vi "Error Converter (ErrCode or Status).vi"(7 "source":string, 10 "error code":i32, 11 "error in (no error)":errorcluster) -> (3 "error out":errorcluster)   [LabVIEW 2026, in "synnax_clib.lvlib"]
uses:
  synnax_clib.lvlib
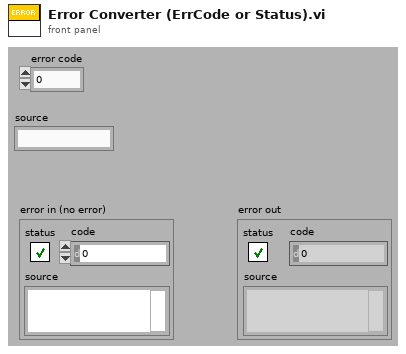
[diagram p1: front panel]
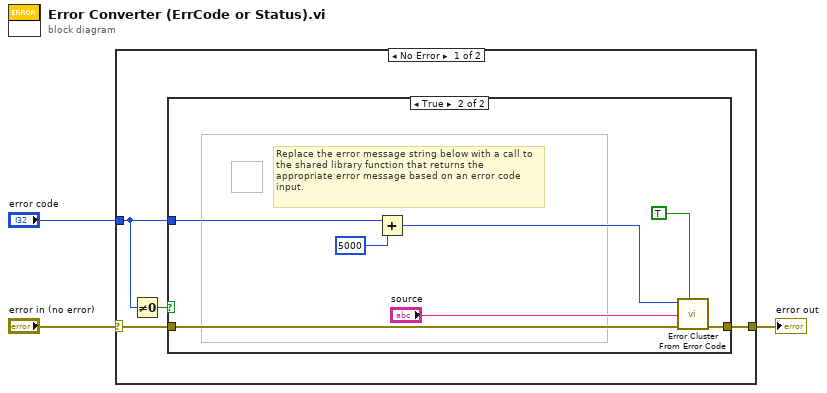
[diagram p0: block diagram]
diagram:
  n1 = case shown="No Error" "error in (no error)" {
    selector: "error in (no error)" -> [w6 w16]
    tunnel: [w4 w16] -> w2
    tunnel: "error code" -> [w5 _]
    frame No Error {
      n2 = Not Equal To 0?(x=w5) -> (x != 0?=w7:bool)
      n3 = case shown="True" w7 {
        tunnel: w6 -> [w8 w15]
        tunnel: w5 -> [_ w13]
        tunnel: [w8 w14] -> w4
        frame False {
        }
        frame True {
          # "Replace the error message string below with a call to the shared library function that returns the appropriate error message based on an error code input."
          n4 = Add(x=w13, y=5000) -> (x+y=w10:i32)
          n5 = call <vilib>:"Error Cluster From Error Code.vi"("show call chain? (False)"=TRUE, "error in (no error)"=w15, "error message (\"\")"="source", "error code (0)"=w10) -> ("error out"=w14:errorcluster)  [unwired: 5 in]
        }
      }
    }
    frame Error {
    }
  }
  "error out" <- w2
